vi "Update_Reference.vi"(6 "Skip Update?":bool, 8 "error in (no error)":errorcluster, 9 "StatusWord":u16, 10 "ControlWord":u16 format="%.0b", 11 "SoftmotionAxis in":refnum<class "SoftmotionAxis.lvclass">) -> (0 "error out":errorcluster, 1 "StatusWord Out":u16, 3 "SoftmotionAxis out":refnum<class "SoftmotionAxis.lvclass">)   [LabVIEW 2017, in "SoftmotionAxis.lvclass"]
uses:
  SoftmotionAxis.lvclass
  <resource>/objmgr/nimotion.rc
  Utilities/Bit Manipulation.lvlib
  <resource>/objmgr/nimcai.rc
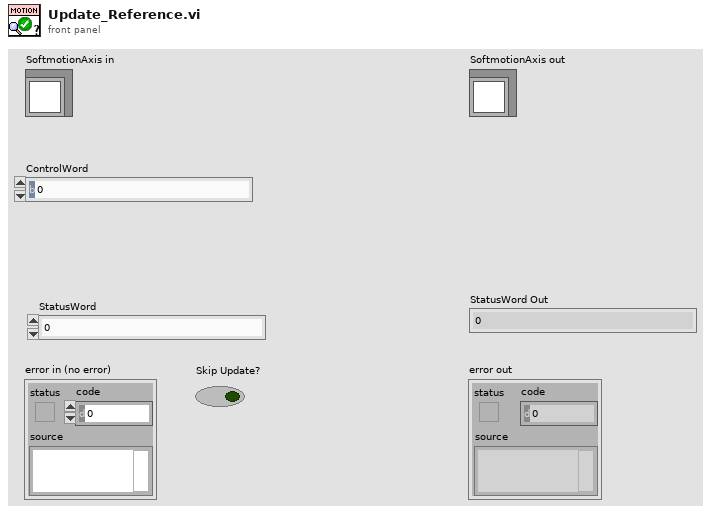
[diagram p1: front panel]
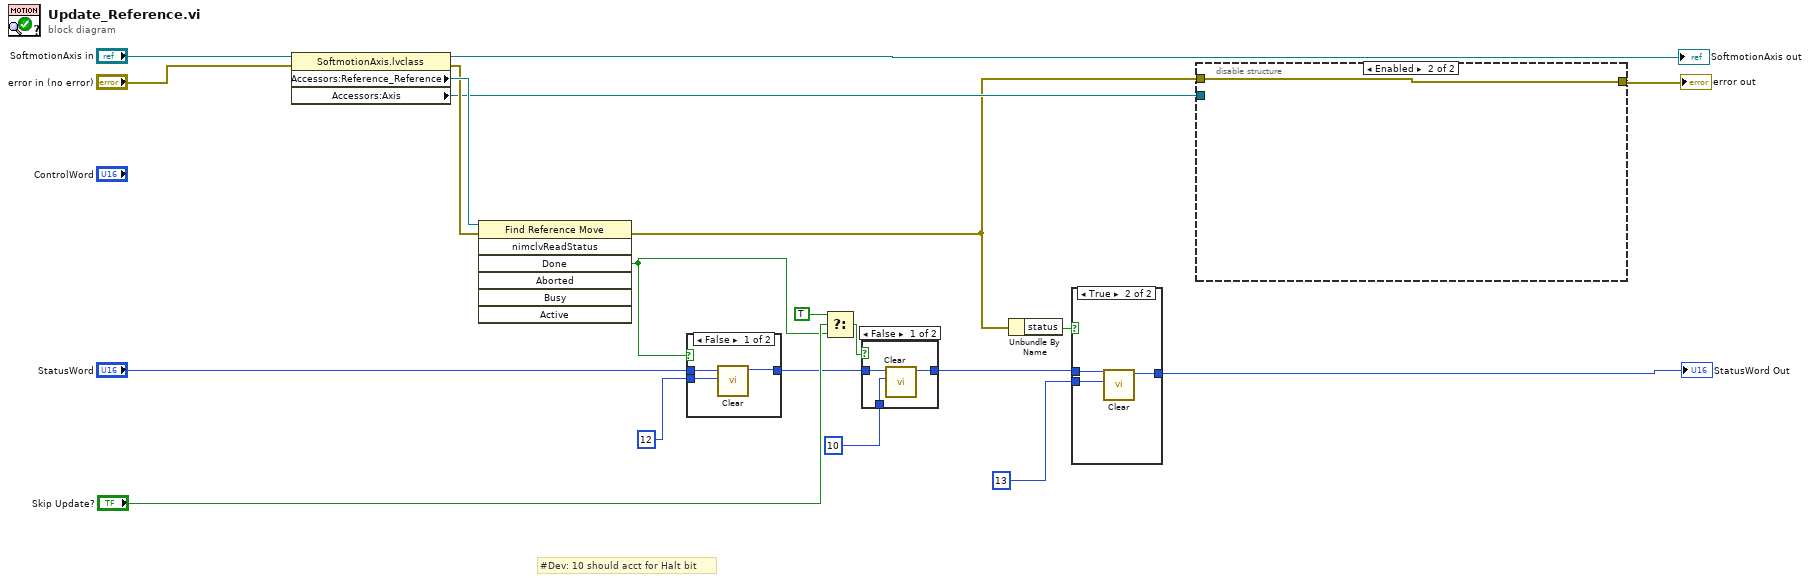
[diagram p0: block diagram]
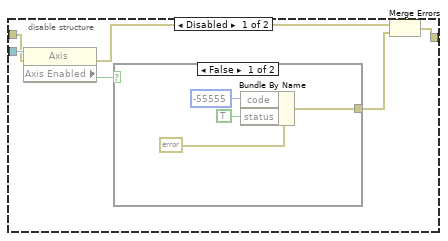
[diagram p2: hidden frame]
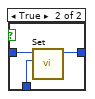
[diagram p4: hidden frame]
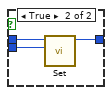
[diagram p5: hidden frame]
diagram:
  # "#Dev: 10 should acct for Halt bit"
  n1 = property class="SoftmotionAxis.lvclass"(reference="SoftmotionAxis in", error in="error in (no error)") -> (reference out=→"SoftmotionAxis out":refnum<class "SoftmotionAxis.lvclass">, error out=w12:errorcluster, "Accessors:Reference_Reference"=w13:refnum<k20>, "Accessors:Axis"=w7:refnum<k21>)
  n2 = invoke class="Find Reference Move" method="nimclvReadStatus"(reference=w13, error in=w12) -> (error out=w5:errorcluster, "Done"=w3:bool)  [unwired: 5 in, 5 out]
  n3 = case shown="False" w3 {
    tunnel: u8 12 -> [w23 w26]
    tunnel: "StatusWord" -> [w22 w25]
    tunnel: [w21 w24] -> w4
    frame False {
      n4 = call "Clear.vi"("Bit to clear"=w23, "Data_In"=w22) -> ("Data_Out"=w21:u16)  [unwired: 9 in]
    }
    frame True {
      n5 = call "Set.vi"("Bit to set"=w26, "Data_In"=w25) -> ("Data_Out"=w24:u16)  [unwired: 9 in]
    }
  }
  n6 = Select(t=TRUE, s="Skip Update?", f=w3) -> (s? t:f=w1:bool)
  n7 = case shown="False" w1 {
    tunnel: [w28 w32] -> w10
    tunnel: u8 10 -> [w27 w31]
    tunnel: w4 -> [w29 w30]
    frame False {
      n8 = call "Clear.vi"("Bit to clear"=w27, "Data_In"=w29) -> ("Data_Out"=w28:u16)  [unwired: 9 in]
    }
    frame True {
      n9 = call "Set.vi"("Bit to set"=w31, "Data_In"=w30) -> ("Data_Out"=w32:u16)  [unwired: 9 in]
    }
  }
  n10 = Unbundle By Name(w5) -> ("status"=w9:bool)
  n11 = case shown="True" w9 {
    tunnel: w10 -> [w33 w36]
    tunnel: [w33 w35] -> w15
    tunnel: u8 13 -> [_ w34]
    frame False {
    }
    frame True {
      n12 = call "Clear.vi"("Bit to clear"=w34, "Data_In"=w36) -> ("Data_Out"=w35:u16)  [unwired: 9 in]
    }
  }
  "StatusWord Out" <- w15
  n13 = disable-structure shown="Enabled" {
    disable-tunnel: [w39 w47] -> w19
    disable-tunnel: w7 -> [w38 _]
    disable-tunnel: w5 -> [w37 w47]
    frame Disabled {
      n14 = property class="Axis"(reference=w38, error in=w37) -> (error out=w40:errorcluster, "Axis Enabled"=w42:bool)  [unwired: 1 out]
      n15 = case shown="False" w42 {
        tunnel: [w43 _] -> w41
        frame False {
          n16 = Bundle By Name(cluster=errorcluster {"status"=FALSE, "code"=0, "source"=""} ("error in (no error)"), "code"=-55555, "status"=TRUE) -> (w43:errorcluster)
        }
        frame True {
        }
      }
      n17 = Merge Errors(w40, w41) -> (w39:errorcluster)
    }
    frame Enabled {
    }
  }
  "error out" <- w19
